vi "Model--Set Value by Name.vi"(8 "error in":errorcluster, 10 "Name":string, 11 "Selector in":refnum<class "Selector.lvclass">) -> (0 "error out":errorcluster, 2 "element":T1, 3 "Selector out":refnum<class "Selector.lvclass">)   [LabVIEW 2019, in "Selector.lvclass"]
uses:
  Selector.lvclass
  Item.ctl
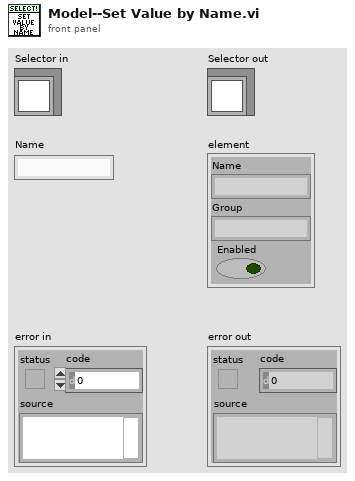
[diagram p1: front panel]
types:
  T1 = typedef "Selector.lvclass/Item.ctl" = cluster{"Name":string, "Group":string, "Enabled":bool}
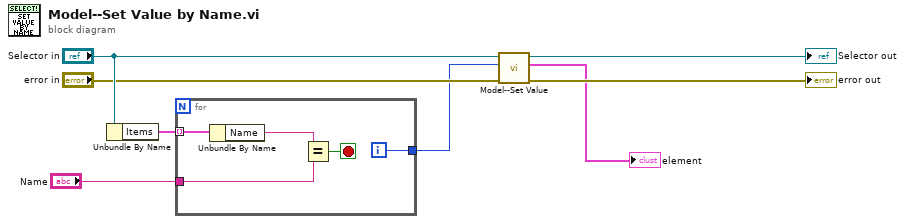
[diagram p0: block diagram]
diagram:
  n1 = Unbundle By Name("Selector in") -> ("Items"=w8:T1[])
  n2 = for {
    tunnel: w8 -> [w13] mode=indexing
    tunnel: "Name" -> [w11]
    tunnel: [w9] -> w2
    i -> [w9]
    stop <- w10 stop-if-true
    n3 = Unbundle By Name(w13) -> ("Name"=w12:string)
    n4 = Equal?(x=w12, y=w11) -> (x = y?=w10:bool)
  }
  n5 = call "Model--Set Value.vi"("error in"="error in", "Value"=w2, "Selector in"="Selector in") -> ("error out"=→"error out":errorcluster, "element"=→"element":T1, "Selector out"=→"Selector out":refnum<class "Selector.lvclass">)  [unwired: 6 in]
